vi "Create Plot Object.vi"(6 "Control Ref Queue":T1, 7 "Actual Transform In":T2, 8 "error in (no error)":errorcluster, 9 "Multiplot Representation In":T4, 10 "3D Ribbon.lvclass in":refnum<class "3D Ribbon.lvclass">, 11 "Plot Object In":refnum<vi>) -> (0 "error out":errorcluster, 1 "Multiplot Representation Out":T4, 2 "3D Ribbon.lvclass out":refnum<class "3D Ribbon.lvclass">, 3 "Plot Object Out":refnum<vi>, 5 "Actual Transform Out":T2)   [LabVIEW 2020, in "3D Ribbon.lvclass"]
uses:
  <vilib>/Math Plots/3D Math Plots/3D Ribbon/3D Ribbon/3D Ribbon.lvclass
  <vilib>/Math Plots/3D Math Plots/3D Plot/3D Plot/Typedef/Multiplot Representation.ctl
  <vilib>/Math Plots/3D Math Plots/3D Plot/3D Plot/Typedef/Plot Representation.ctl
  <vilib>/Math Plots/3D Math Plots/3D Plot/3D Plot/Typedef/Range Clusters.ctl
  <vilib>/Math Plots/3D Math Plots/3D Plot/3D Plot/Typedef/Mesh Data.ctl
  <vilib>/Math Plots/3D Math Plots/3D Plot/3D Plot/Typedef/Actual Transform.ctl
  <vilib>/Math Plots/3D Math Plots/3D Plot/Action String/3DMathPlot Ctrl Act Queue.ctl
  <vilib>/Math Plots/3D Math Plots/3D Plot/Action String/3DMathPlot Ctrl Act Cluster.ctl
  <vilib>/Math Plots/3D Math Plots/3D Plot/Action String/3DMathPlot State Class.ctl
  <vilib>/Math Plots/3D Math Plots/3D Ribbon/3D Ribbon/3D Ribbon.lvclass/3D Ribbon.ctl
  <vilib>/Math Plots/3D Math Plots/3D Plot/3D Plot/3D Plot.lvclass
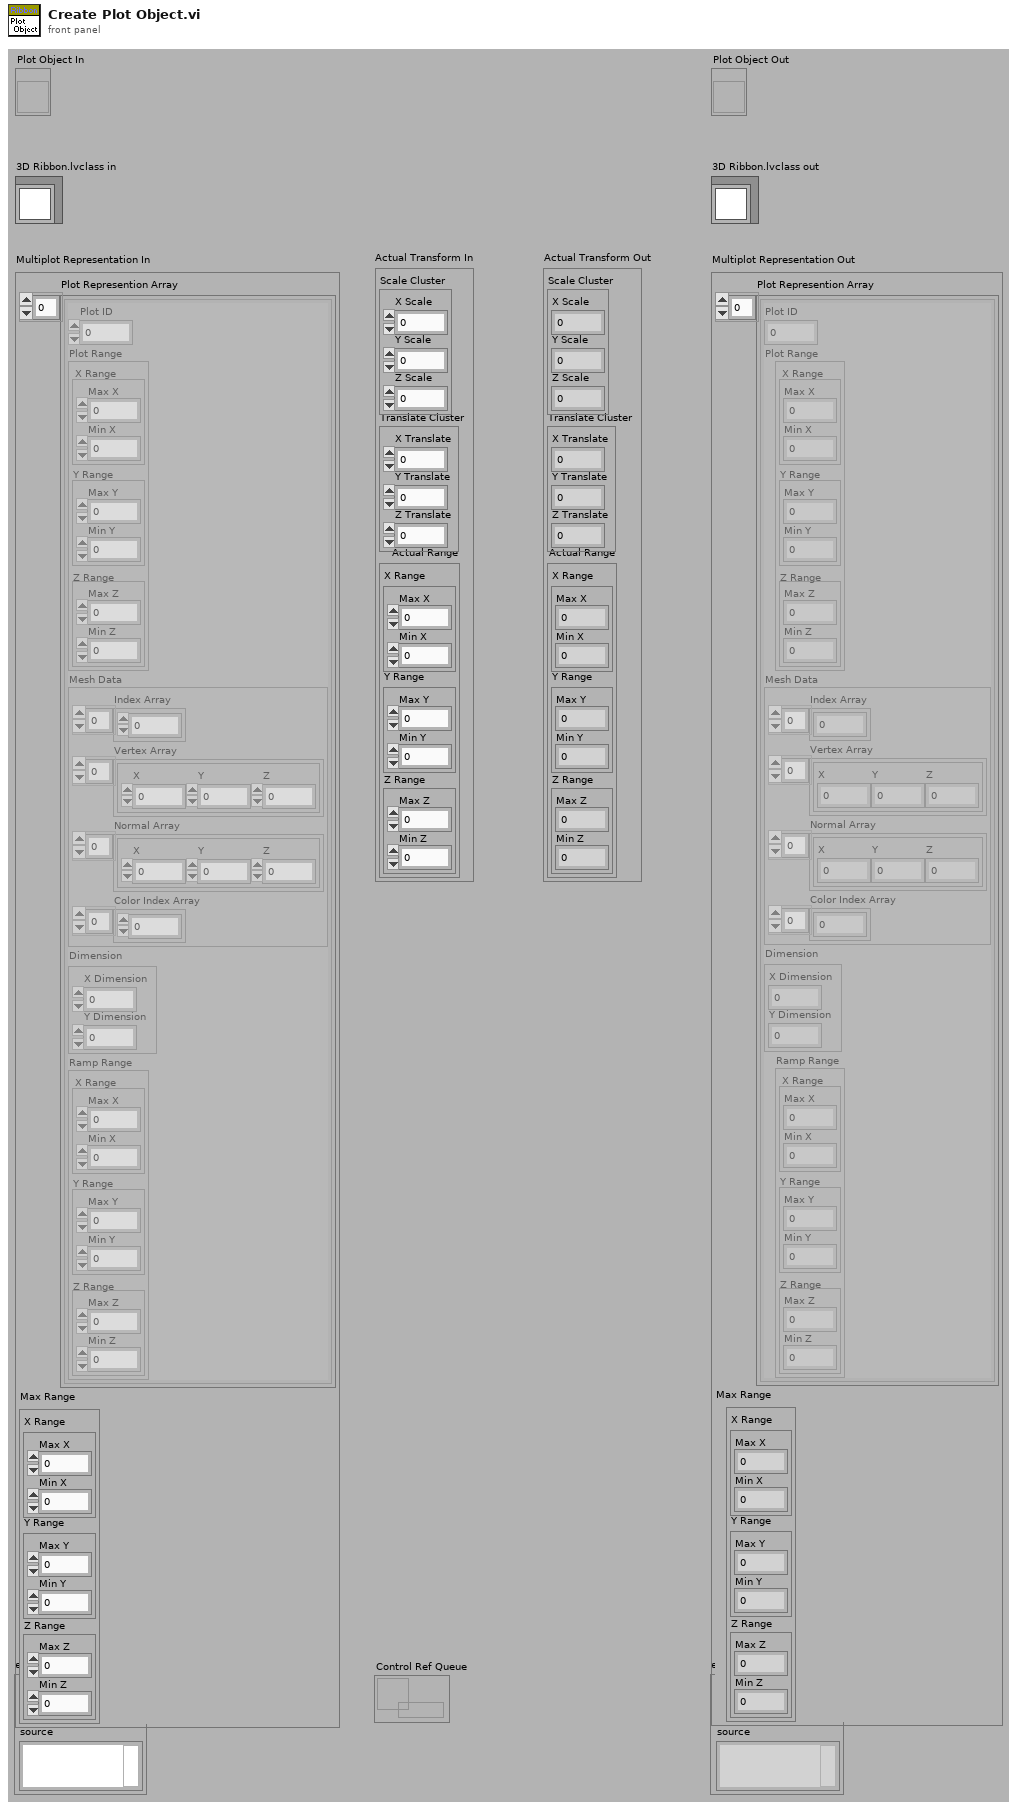
[diagram p1: front panel]
types:
  T1 = typedef "3DMathPlot Ctrl Act Queue.ctl" = refnum<queue>
  T2 = typedef "3D Plot.lvclass/Actual Transform.ctl" = cluster{"Scale Cluster":cluster{"X Scale":sgl, "Y Scale":sgl, "Z Scale":sgl}, "Translate Cluster":cluster{"X Translate":sgl, "Y Translate":sgl, "Z Translate":sgl}, "Actual Range":T3}
  T3 = typedef "3D Plot.lvclass/Range Clusters.ctl" = cluster{"X Range":cluster{"Max X":sgl, "Min X":sgl}, "Y Range":cluster{"Max Y":sgl, "Min Y":sgl}, "Z Range":cluster{"Max Z":sgl, "Min Z":sgl}}
  T4 = typedef "3D Plot.lvclass/Multiplot Representation.ctl" = cluster{"Plot Represention Array":T5[], "Max Range":T3}
  T5 = typedef "3D Plot.lvclass/Plot Representation.ctl" = cluster{"Plot ID":i32, "Plot Range":T3, "Mesh Data":T6, "Dimension":cluster{"X Dimension":i32, "Y Dimension":i32}, "Ramp Range":T3}
  T6 = typedef "3D Plot.lvclass/Mesh Data.ctl" = cluster{"Index Array":u32[], "Vertex Array":cluster{"X":sgl, "Y":sgl, "Z":sgl}[], "Normal Array":cluster{"X":sgl, "Y":sgl, "Z":sgl}[], "Color Index Array":i32[]}
  T7 = typedef "3D Ribbon.lvclass/3D Ribbon Property Array.ctl" = T8[]
  T8 = typedef "3D Ribbon.lvclass/3D Ribbon Property.ctl" = cluster{"General Property":cluster{"Plot Name":string, "Coordinate System":enum16{"Cartesian", "Cylindrical", "Spherical"}, "Opacity":sgl}, "Projection Property":cluster{"Draw XY":bool, "Draw YZ":bool, "Draw XZ":bool}, "Plot Property":cluster{"Draw Surface":bool, "Color Ramp Cluster":T9, "Line Style":T10, "Line Width":sgl, "Line Color":u32, "Antialiasing":bool}, "Ribbon Property":cluster{"Ribbon Mode":enum16{"Row", "Column"}, "Ribbon Width":sgl}}
  T9 = typedef "3D Plot.lvclass/Color Ramp Cluster.ctl" = cluster{"Color Ramp Style":enum16{"None", "Shaded", "Color spectrum", "Grey scale", "Custom"}, "Color Ramp Array":u32[], "Color Ramp Index":i32[], "Interpolate?":bool, "Logarithm?":bool}
  T10 = typedef "3D Plot.lvclass/Line Type.ctl" = enum16{"None", "Solid", "Dash", "Dot", "Dash Dot"}
  T11 = enum16{"Points", "Lines", "Line Strip", "Line Loop", "Triangles", "Triangle Strip", "Triangle Fan", "Quads", "Quad Strip", "Polygon"}
  T12 = cluster{"Draw XY":bool, "Draw YZ":bool, "Draw XZ":bool}
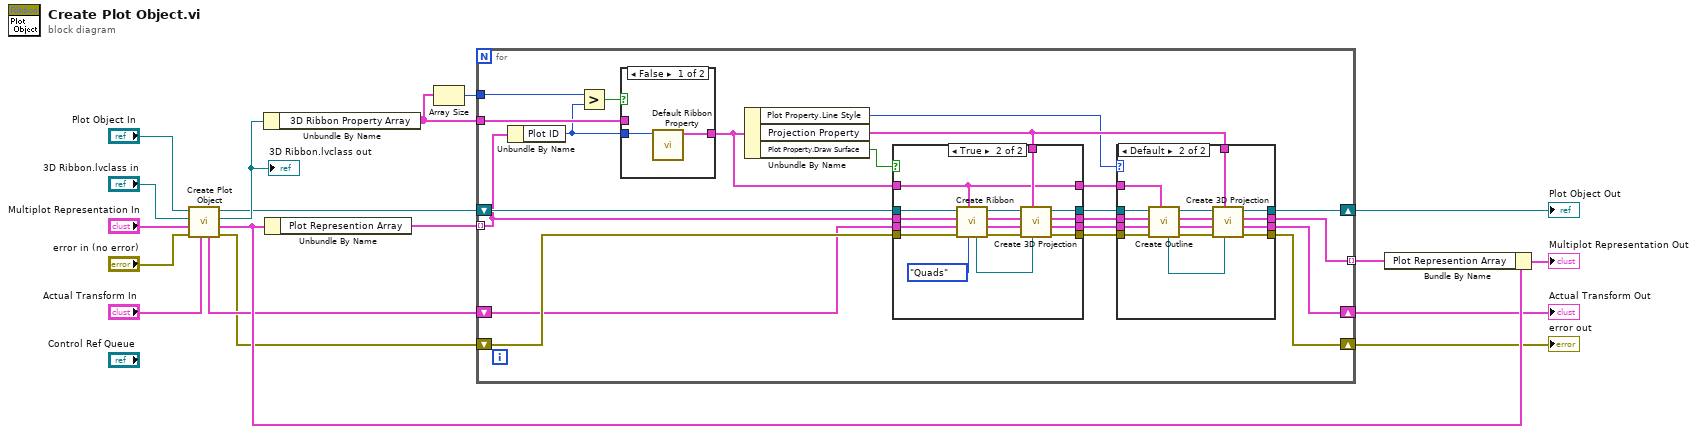
[diagram p0: block diagram]
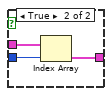
[diagram p2: hidden frame]
diagram:
  n1 = call-parent "Create Plot Object.vi"("Actual Transform In"="Actual Transform In", "error in (no error)"="error in (no error)", "Multiplot Representation In"="Multiplot Representation In", "3D Plot.lvclass in"="3D Ribbon.lvclass in", "Plot Object In"="Plot Object In") -> ("error out"=w5:errorcluster, "Multiplot Representation Out"=w11:T4, "3D Plot.lvclass out"=w6:refnum<class "3D Ribbon.lvclass">, "Plot Object Out"=w4:refnum<vi>, "Actual Transform Out"=w10:T2)  [unwired: 1 in, 1 out]
  "3D Ribbon.lvclass out" <- w6
  n2 = Unbundle By Name(w6) -> ("3D Ribbon Property Array"=w2:T7)
  n3 = Unbundle By Name(w11) -> ("Plot Represention Array"=w13:T5[])
  n4 = Array Size(array=w2) -> (size(s)=w1:i32)
  n5 = for {
    shift-right: [w37] -> w7
    shift-left: w5 -> [w34]
    shift-right: [w39] -> w3
    shift-left: w4 -> [w36]
    shift-right: [w38] -> w8
    shift-left: w10 -> [w29]
    tunnel: w13 -> [w35] mode=indexing
    tunnel: [w27] -> w12 mode=indexing
    tunnel: w2 -> [w20]
    tunnel: w1 -> [w22]
    n6 = Unbundle By Name(w35) -> ("Plot ID"=w19:i32)
    n7 = Greater?(x=w22, y=w19) -> (0:w23:bool)
    n8 = case shown="False" w23 {
      tunnel: w20 -> [_ w44]
      tunnel: [w41 w43] -> w21
      tunnel: w19 -> [w40 w42]
      frame False {
        n9 = call <vilib>:"Default Ribbon Property.vi"("Plot ID"=w40) -> ("Default Property"=w41:T8)  [unwired: 10 out]
      }
      frame True {
        n10 = Index Array(array=w44, index=w42) -> (element=w43:T8)
      }
    }
    n11 = Unbundle By Name(w21) -> ("Plot Property.Line Style"=w24:T10, "Projection Property"=w33:T12, "Plot Property.Draw Surface"=w25:bool)
    n12 = case shown="True" w25 {
      tunnel: w36 -> [w65 w80]
      tunnel: w35 -> [w64 w79]
      tunnel: w34 -> [w62 w75]
      tunnel: w33 -> [_ w74]
      tunnel: w21 -> [w66 w67]
      tunnel: [w65 w72] -> w32
      tunnel: [w62 w71] -> w31
      tunnel: [w63 w70] -> w30
      tunnel: w29 -> [w63 w69]
      tunnel: [w64 w68] -> w28
      tunnel: [w66 w67] -> w26
      frame False {
      }
      frame True {
        n13 = call <vilib>:"Create Ribbon.vi"("Draw Mode"=T11."Quads", "3D Ribbon Property"=w67, "error in (no error)"=w75, "Plot Representation In"=w79, "Plot Object In"=w80) -> ("error out"=w78:errorcluster, "Plot Representation Out"=w68:T5, "Plot Object Out"=w77:refnum<vi>, "Ribbon Object Out"=w76:refnum<vi>)  [unwired: 2 in, 1 out]
        n14 = call <vilib>:"Create 3D Projection.vi"("Sub Object In"=w76, "Projection Property"=w74, "error in (no error)"=w78, "Actual Transform In"=w69, "Plot Object In"=w77) -> ("error out"=w71:errorcluster, "Actual Transform Out"=w70:T2, "Plot Object Out"=w72:refnum<vi>)  [unwired: 1 in, 3 out]
      }
    }
    n15 = case shown="Default" w24 {
      tunnel: [w48 w61] -> w39
      tunnel: [w46 w60] -> w38
      tunnel: [w45 w59] -> w37
      tunnel: w33 -> [_ w58]
      tunnel: w26 -> [_ w57]
      tunnel: w32 -> [w48 w56]
      tunnel: w31 -> [w45 w54]
      tunnel: w30 -> [w46 w52]
      tunnel: w28 -> [w47 w50]
      tunnel: [w47 w49] -> w27
      frame "None" {
      }
      frame Default {
        n16 = call <vilib>:"Create Outline.vi"("3D Ribbon Property"=w57, "error in (no error)"=w54, "Plot Representation In"=w50, "Plot Object In"=w56) -> ("error out"=w53:errorcluster, "Plot Representation Out"=w49:T5, "Plot Object Out"=w55:refnum<vi>, "Outline Object Out"=w51:refnum<vi>)  [unwired: 4 out]
        n17 = call <vilib>:"Create 3D Projection.vi"("Sub Object In"=w51, "Projection Property"=w58, "error in (no error)"=w53, "Actual Transform In"=w52, "Plot Object In"=w55) -> ("error out"=w59:errorcluster, "Actual Transform Out"=w60:T2, "Plot Object Out"=w61:refnum<vi>)  [unwired: 1 in, 3 out]
      }
    }
  }
  "error out" <- w7
  "Plot Object Out" <- w3
  "Actual Transform Out" <- w8
  n18 = Bundle By Name(cluster=w11, "Plot Represention Array"=w12) -> (→"Multiplot Representation Out":T4)
